vi "XY Plot Matrix.vi"() -> ()   [LabVIEW 2020]
doc: "This VI shows how to use the XY Plot Matrix indicator."
uses:
  <vilib>/Math Plots/2D Math Plots/XY Plot Matrix/XY Plot Matrix XCtrl/XY Plot Matrix.xctl
  <vilib>/Math Plots/2D Math Plots/XY Plot Matrix/XY Plot Matrix Datatype/XY Plot Matrix Datatype.lvclass
panel:
  out "XY Plot Matrix":refnum<class "XY Plot Matrix Datatype.lvclass">[](xcontrol)
  # "Overview: Demonstrates the XY Plot Matrix indicator.\nInstructions:\nRun the VI."
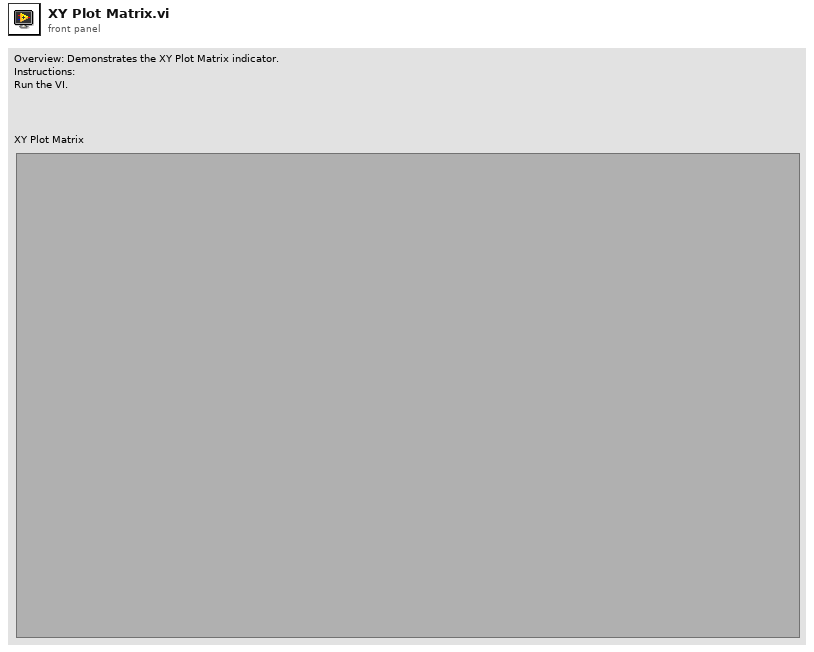
[diagram p1: front panel]
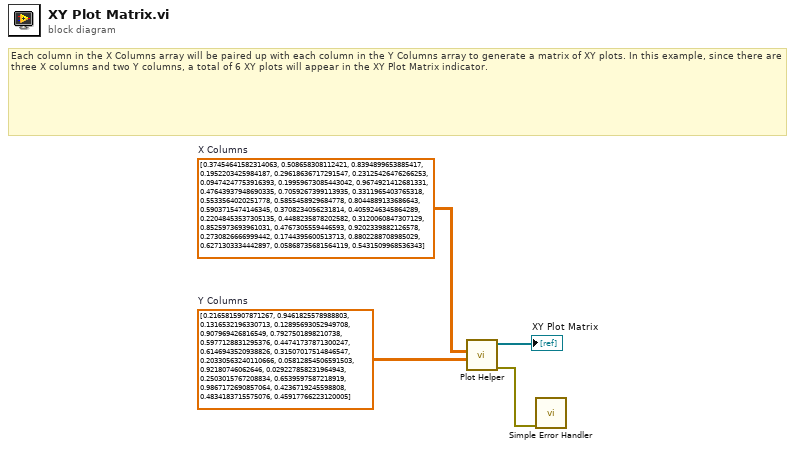
[diagram p0: block diagram]
diagram:
  w4 = dbl[][] [[0.37454641582314063, 0.508658308112421, 0.8394899653885417], [0.1952203425984187, 0.29618636717291547, 0.23125426476266253], [0.09474247753916393, 0.19959673085443042, 0.9674921412681331], [0.47643937948690335, 0.7059267399113935, 0.3311965403765318], [0.5533564020251778, 0.5855458929684778, 0.8044889133686643], [0.5903715474146345, 0.3708234056231814, 0.4059246345864289], [0.22048453537305135, 0.4488235878202582, 0.3120060847307129], [0.8525973693961031, 0.4767305559446593, 0.9202339882126578], [0.2730826666999442, 0.1744395600513713, 0.8802288708985029], [0.6271303334442897, 0.05868735681564119, 0.5431509968536343]]  # X Columns
  w3 = dbl[][] [[0.2165815907871267, 0.9461825578988803], [0.1316532196330713, 0.12895693052949708], [0.907969426816549, 0.7927501898210738], [0.5977128831295376, 0.44741737871300247], [0.6146943520938826, 0.31507017514846547], [0.20330563240110666, 0.05812854506591503], [0.92180746062646, 0.029227858231964943], [0.2503015767208834, 0.6539597587218919], [0.9867172690857064, 0.4236719245598808], [0.4834183715575076, 0.45917766223120005]]  # Y Columns
  # "Each column in the X Columns array will be paired up with each column in the Y Columns array to generate a matrix of XY plots. In this example, since there are three X columns and two Y columns, a total of 6 XY plots will appear in the XY Plot Matrix indicator."
  n1 = call <vilib>:"Plot Helper.vi"("y matrix"=w3, "x matrix"=w4) -> ("error out"=w2:errorcluster, "2D Plotmatrix Class Obj Array out"=→"XY Plot Matrix":refnum<class "XY Plot Matrix Datatype.lvclass">[])  [unwired: 2 in, 6 out]
  n2 = call <vilib>:"Simple Error Handler.vi"("error in (no error)"=w2) -> ()  [unwired: 4 in, 5 out]
